vi "SetNotzero (SubVI).vi"(8 "error in (no error)":errorcluster, 9 "Value":sgl, 10 "Control Name":string, 11 "VI in":refnum<vi>) -> (0 "error out":errorcluster, 3 "VI out":refnum<vi>)   [LabVIEW 2014]
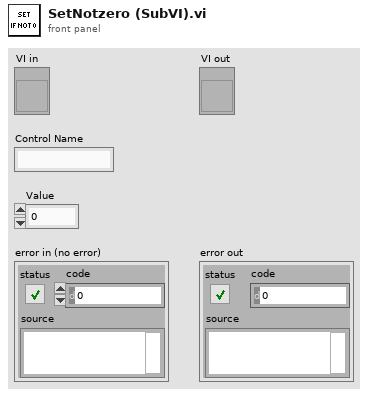
[diagram p1: front panel]
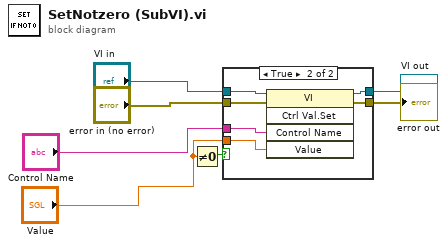
[diagram p0: block diagram]
diagram:
  n1 = Not Equal To 0?(x="Value") -> (x != 0?=w5:bool)
  n2 = case shown="True" w5 {
    tunnel: [w9 w15] -> w1
    tunnel: "VI in" -> [w9 w14]
    tunnel: [w8 w13] -> w3
    tunnel: "error in (no error)" -> [w8 w12]
    tunnel: "Value" -> [_ w11]
    tunnel: "Control Name" -> [_ w10]
    frame False {
    }
    frame True {
      n3 = invoke class="VI" method="Ctrl Val.Set"(reference=w14, error in=w12, "Control Name"=w10, "Value"=w11) -> (reference out=w15:refnum<vi>, error out=w13:errorcluster)  [unwired: 1 in, 3 out]
    }
  }
  "error out" <- w3
  "VI out" <- w1
